vi "Capture@Display2User__Parameter.vi"(1 "ParamterIn":string) -> (0 "ParamterOut":string)   [LabVIEW 2020]
panel:
  in  "RefName":string(combo)
  in  "CamName":string(combo)
  in  "Confirm":bool
  # "Capture@Display2User $Capture,$UserPanelControlName"
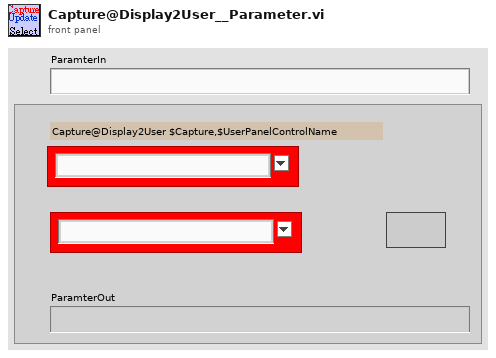
[diagram p1: front panel]
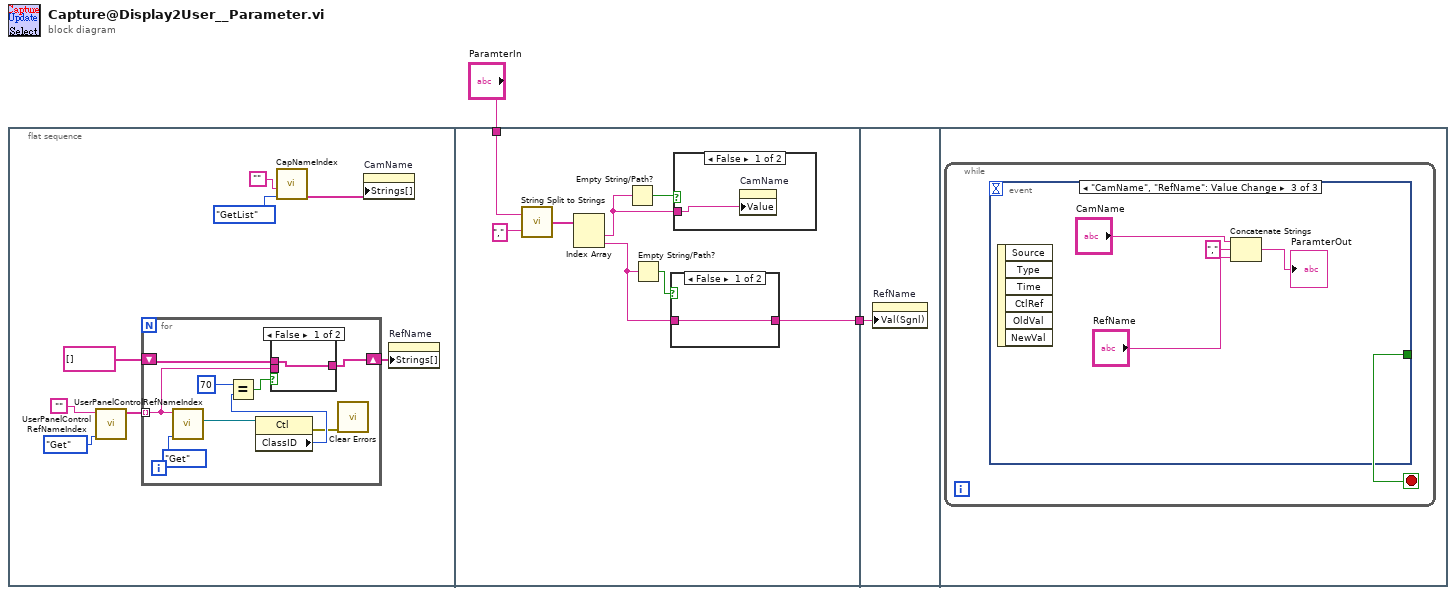
[diagram p0: block diagram]
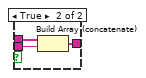
[diagram p2: hidden frame]
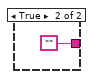
[diagram p3: hidden frame]
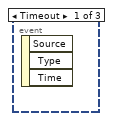
[diagram p5: hidden frame]
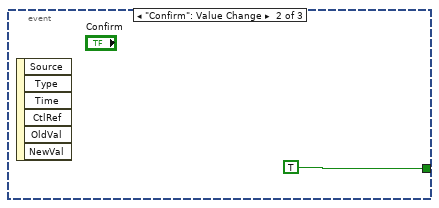
[diagram p6: hidden frame]
diagram:
  n1 = flat-sequence {
    tunnel: "ParamterIn" -> [w27]
    tunnel: [w24] -> w1
    tunnel: w1 -> [w35]
    frame #0 {
      n2 = call "UserPanelControlRefNameIndex.vi"("OP"=enum16{"Get", "Update", "Init"}."Get", "ControlName"="") -> ("ControlNameS"=w7:string[])  [unwired: 6 in, 3 out]
      n3 = for {
        tunnel: w7 -> [w14] mode=indexing
        shift-right: [w13] -> w3
        shift-left: string[] [] ("Strings []") -> [w15]
        n4 = call "UserPanelControlRefNameIndex.vi"("OP"=enum16{"Get", "Update", "Init"}."Get", "ControlName"=w14) -> ("ControlRefOut"=w18:refnum<vi>)  [unwired: 6 in, 3 out]
        n5 = property class="Ctl"(reference=w18) -> (error out=w11:errorcluster, "ClassID"=w17:u32)  [unwired: 1 in, 1 out]
        n6 = Equal?(x=u32 70, y=w17) -> (x = y?=w16:bool)
        n7 = case shown="False" w16 {
          tunnel: w15 -> [w20 w23]
          tunnel: w14 -> [_ w22]
          tunnel: [w20 w21] -> w13
          frame False {
          }
          frame True {
            n8 = Build Array (concatenate)(w23, w22) -> (w21:string[])
          }
        }
        n9 = call <vilib>:"Clear Errors.vi"("error in (no error)"=w11) -> ()  [unwired: 5 in, 2 out]
      }
      n10 = call "CapNameIndex.vi"("OP"=enum16{"AddCam", "GetIndex", "Init", "GetList"}."GetList", "CamName"="") -> ("DeviceList"=w9:string[])  [unwired: 2 in, 3 out]
      n11 = property on="CamName" class="CmbBox"("Strings[]"=w9) -> ()  [unwired: 2 in, 2 out]
      n12 = property on="RefName" class="CmbBox"("Strings[]"=w3) -> ()  [unwired: 2 in, 2 out]
    }
    frame #1 {
      n13 = call "String Split to Strings.vi"("search string/char (-)"=",", "String"=w27) -> ("Array"=w28:string[])
      n14 = Index Array(array=w28) -> (element #1=w26:string, element #2=w25:string)  [unwired: 2 in]
      n15 = Empty String/Path?(string/path=w26) -> (empty?=w31:bool)
      n16 = Empty String/Path?(string/path=w25) -> (empty?=w30:bool)
      n17 = case shown="False" w30 {
        tunnel: [w32 ""] -> w24
        tunnel: w25 -> [w32 _]
        frame False {
        }
        frame True {
        }
      }
      n18 = case shown="False" w31 {
        tunnel: w26 -> [w34 _]
        frame False {
          n19 = property on="CamName" class="CmbBox"("Value"=w34) -> ()  [unwired: 2 in, 2 out]
        }
        frame True {
        }
      }
    }
    frame #2 {
      n20 = property on="RefName" class="CmbBox"("Val(Sgnl)"=w35) -> ()  [unwired: 2 in, 2 out]
    }
    frame #3 {
      n21 = while {
        stop <- w36 stop-if-true
        n22 = event shown="[2] \"CamName\", \"RefName\": Value Change" {
          selector: _ -> [_ _ _]
          dyn-events: _ -> [_ _ _]
          timeout: _ -> [_ _ _]
          tunnel: [_ TRUE _] -> w36
          event Timeout {
            n23 = event-data() -> ()  [unwired: 1 in, 3 out]
          }
          event "Confirm": Value Change {
            n24 = event-data() -> ()  [unwired: 1 in, 6 out]
          }
          event "CamName", "RefName": Value Change {
            n25 = event-data() -> ()  [unwired: 1 in, 6 out]
            n26 = Concatenate Strings("CamName", "," ("string"), "RefName") -> (→"ParamterOut":string)
          }
        }
      }
    }
  }
